vi "xcorr.bkp.vi"(4 "shift":u8, 6 "N":u8, 7 "y":u32, 8 "x":u32, 9 "enable":bool, 10 "lag":u16) -> (1 "Rxy valid":bool, 2 "Rxy":u64, 3 "trigger":bool)   [LabVIEW 2017]
uses:
  <vilib>/rvi/FXPMathLib/basic elements/FxpDiscreteDelay/XNode/nifxpmath_DiscreteDelay.xnode
panel:
  out "Rxy 2":u64
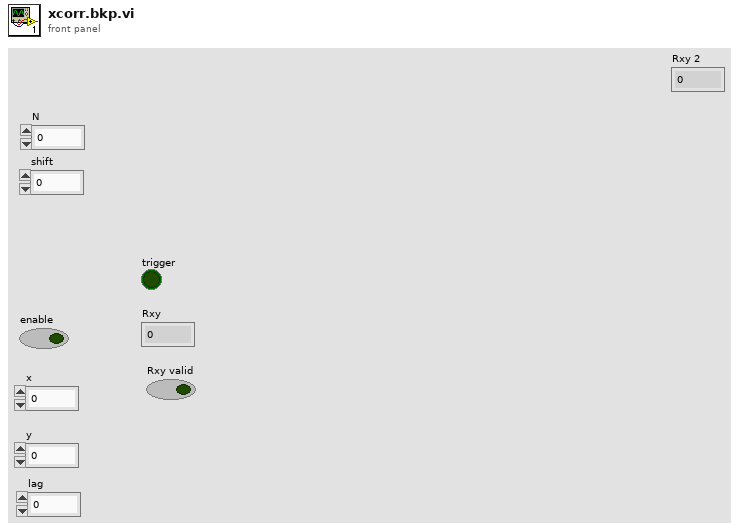
[diagram p1: front panel]
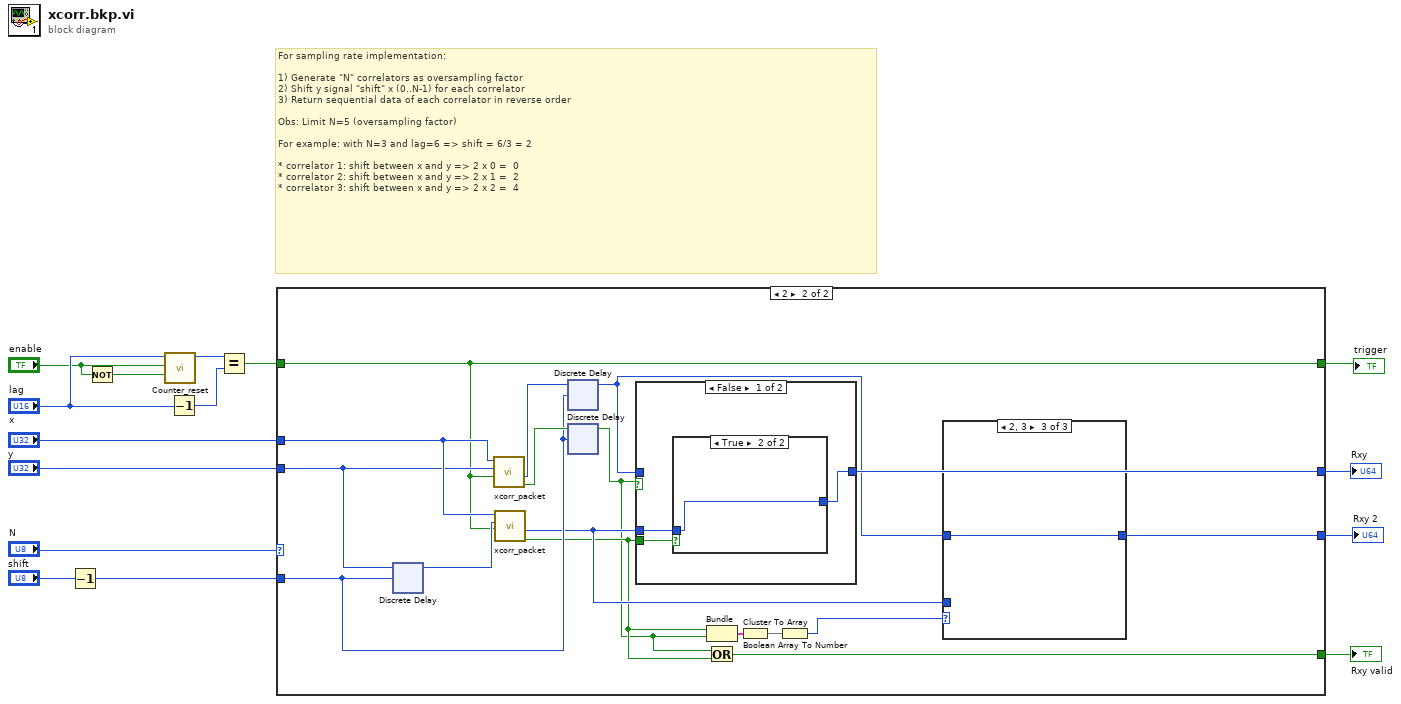
[diagram p0: block diagram]
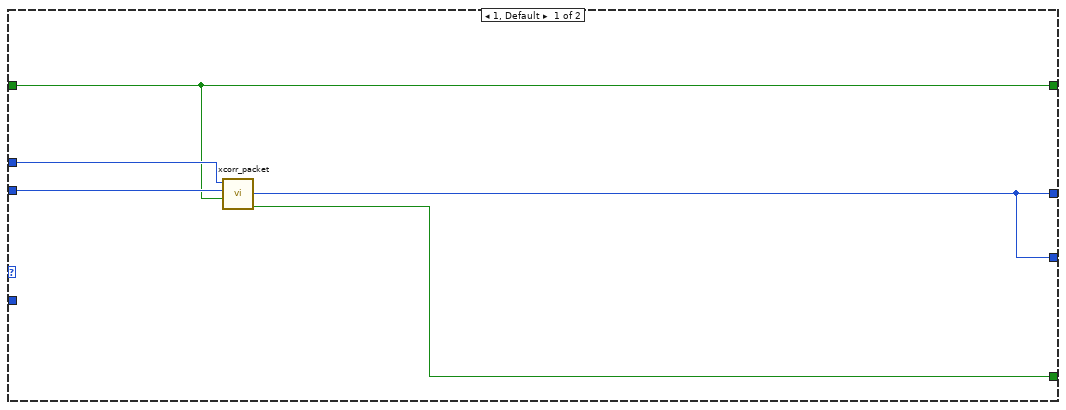
[diagram p2: hidden frame]
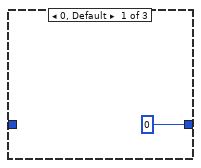
[diagram p3: hidden frame]
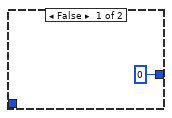
[diagram p5: hidden frame]
diagram:
  # "For sampling rate implementation:\n\n1) Generate \"N\" correlators as oversampling factor\n2) Shift y signal \"shift\" x (0..N-1) for each correlator\n3) Return sequential data of each correlator in reverse order\n\nObs: Limit N=5 (oversampling factor)\n\nFor example: with N=3 and lag=6 => shift = 6/3 = 2\n\n* correlator 1: shift between x and y => 2 x 0 =  0\n* correlator 2: shift between x and y => 2 x 1 =  2\n* correlator 3: shift between x and y => 2 x 2 =  4"
  n1 = Decrement(x="shift") -> (x-1=w8:u8)
  n2 = Not(x="enable") -> (.not. x?=w5:bool)
  n3 = call "Counter_reset.vi"("reset"=w5, "enable"="enable", "limit"="lag") -> ("count"=w7:u16)  [unwired: 8 in]
  n4 = Decrement(x="lag") -> (x-1=w6:u16)
  n5 = Equal?(x=w7, y=w6) -> (x = y?=w4:bool)
  n6 = case shown="2" "N" {
    tunnel: [w16 w36] -> w15
    tunnel: [w20 w35] -> w14
    tunnel: [w17 w29] -> w13
    tunnel: w4 -> [w17 w29]
    tunnel: "x" -> [w19 w37]
    tunnel: "y" -> [w18 w34]
    tunnel: w8 -> [_ w30]
    tunnel: [w16 w25] -> w1
    frame 1, Default {
      n7 = call "xcorr_packet.vi"("x"=w19, "y"=w18, "trigger"=w17) -> ("out"=w16:u64, "valid"=w20:bool)  [unwired: 5 in]
    }
    frame 2 {
      n8 = xnode ("Discrete Delay")("D"=w34, "n-1[0..255]"=w30) -> ("Q"=w33:u32)
      n9 = call "xcorr_packet.vi"("x"=w37, "y"=w34, "trigger"=w29) -> ("out"=w32:u64, "valid"=w31:bool)  [unwired: 5 in]
      n10 = call "xcorr_packet.vi"("x"=w37, "y"=w33, "trigger"=w29) -> ("out"=w23:u64, "valid"=w22:bool)  [unwired: 5 in]
      n11 = xnode ("Discrete Delay")("D"=w32, "n-1[0..255]"=w30) -> ("Q"=w24:u64)
      n12 = xnode ("Discrete Delay")("D"=w31, "n-1[0..255]"=w30) -> ("Q"=w21:bool)
      n13 = case shown="False" w21 {
        tunnel: [w41 w46] -> w36
        tunnel: w24 -> [_ w46]
        tunnel: w22 -> [w43 _]
        tunnel: w23 -> [w42 _]
        frame False {
          n14 = case shown="True" w43 {
            tunnel: [u64 0 ("out") w45] -> w41
            tunnel: w42 -> [_ w45]
            frame False {
            }
            frame True {
            }
          }
        }
        frame True {
        }
      }
      n15 = Bundle("valid"=w22, "Q"=w21) -> (w28:cluster{"valid":bool, "Q":bool})  [unwired: 1 in]
      n16 = Or(x=w21, y=w22) -> (x .or. y?=w35:bool)
      n17 = Cluster To Array(cluster=w28) -> (array=w27:bool[])
      n18 = Boolean Array To Number(Boolean array=w27) -> (number=w26:u8)
      n19 = case shown="2, 3" w26 {
        tunnel: [u64 0 ("out") w39 w40] -> w25
        tunnel: w24 -> [_ _ w40]
        tunnel: w23 -> [_ w39 _]
        frame 0, Default {
        }
        frame 1 {
        }
        frame 2, 3 {
        }
      }
    }
  }
  "trigger" <- w13
  "Rxy valid" <- w14
  "Rxy" <- w15
  "Rxy 2" <- w1
